vi "init_com.vi"(6 "timeout (10sec)":u32=10000, 7 "End Write on Termination Character?":bool, 8 "error in (no error)":errorcluster, 10 "baud rate":u32, 11 "VISA resource name":refnum<visa-resource-name>="COM13") -> (0 "error out":errorcluster)   [LabVIEW 2016, in "BT-Android_interface.lvlib"]
uses:
  BT-Android_interface.lvlib
  mode.ctl
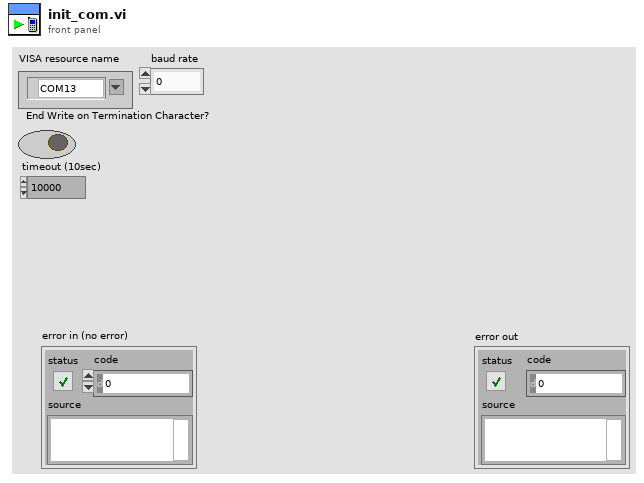
[diagram p1: front panel]
types:
  T1 = typedef "BT-Android_interface.lvlib/mode.ctl" = enum16{"init", "broadcast_data", "receive_data", "close"}
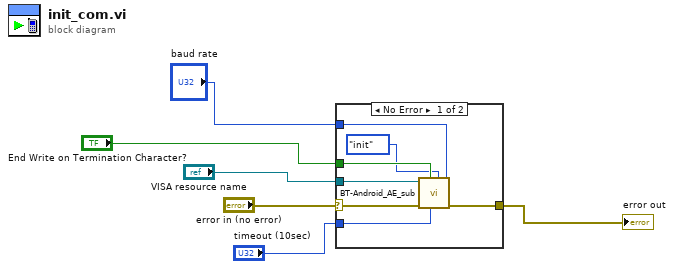
[diagram p0: block diagram]
diagram:
  n1 = case shown="No Error" "error in (no error)" {
    selector: "error in (no error)" -> [w13 w14]
    tunnel: [w12 w14] -> w5
    tunnel: "VISA resource name" -> [w11 _]
    tunnel: "End Write on Termination Character?" -> [w10 _]
    tunnel: "timeout (10sec)" -> [w9 _]
    tunnel: "baud rate" -> [w7 _]
    frame No Error {
      n2 = call "BT-Android_AE_sub.vi"("baud rate"=w7, "mode"=mode."init", "timeout (10sec)"=w9, "End Write on Termination Character?"=w10, "error in (no error)"=w13, "VISA resource name"=w11) -> ("error IO"=w12:errorcluster)  [unwired: 4 in, 1 out]
    }
    frame Error {
    }
  }
  "error out" <- w5
